vi "Do Operations - Use Dynamic Dispatch Method.vi"(8 "error in (no error)":errorcluster, 11 "Array":refnum<class "SimpleArithmetic.lvclass">[](array[class])) -> (0 "error out":errorcluster, 3 "Array Out":refnum<class "SimpleArithmetic.lvclass">[](array[class]))   [LabVIEW 2012]
uses:
  ClassDefinitions/SimpleClassWithMethods/SimpleArithmetic.lvclass
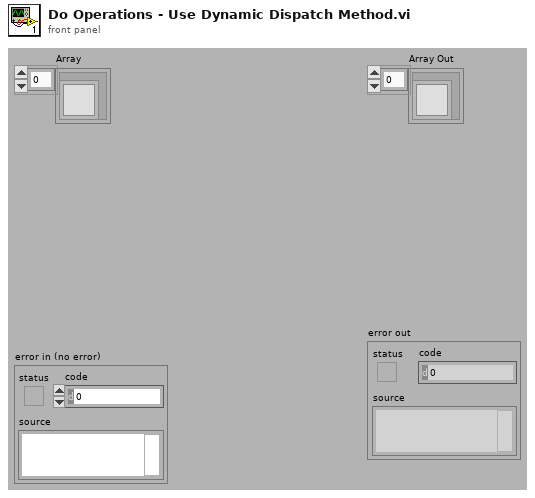
[diagram p1: front panel]
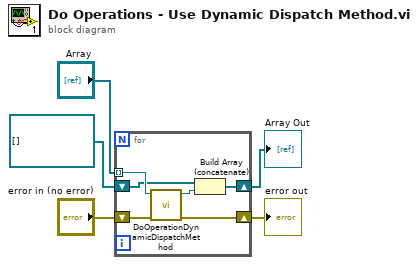
[diagram p0: block diagram]
diagram:
  n1 = for {
    tunnel: "Array" -> [w11] mode=indexing
    shift-right: [w6] -> w1
    shift-left: refnum<class "SimpleArithmetic.lvclass">[] [] ("Array") -> [w9]
    shift-right: [w7] -> w2
    shift-left: "error in (no error)" -> [w10]
    n2 = call-dynamic "DoOperationDynamicDispatchMethod.vi"("error in (no error)"=w10, "SimpleArithmetic in"=w11) -> ("error out"=w7:errorcluster, "SimpleArithmetic out"=w8:refnum<class "SimpleArithmetic.lvclass">)  [unwired: 8 in]
    n3 = Build Array (concatenate)(w9, w8) -> (w6:refnum<class "SimpleArithmetic.lvclass">[])
  }
  "Array Out" <- w1
  "error out" <- w2
